vi "Flush Buffer.vi"(0 "VISA resource name":refnum<visa-resource-name>, 7 "milliseconds to wait":u32, 11 "error in (no error)":errorcluster) -> (4 "VISA resource name out":refnum<visa-resource-name>, 6 "read buffer":string, 8 "return count":u32, 10 "Number of Bytes at Serial Port":u32, 15 "error out":errorcluster)   [LabVIEW 2020]
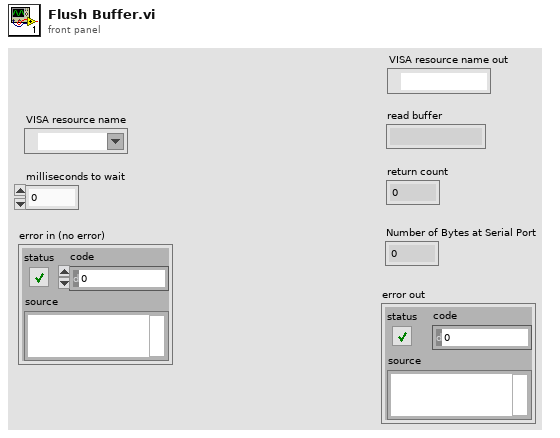
[diagram p1: front panel]
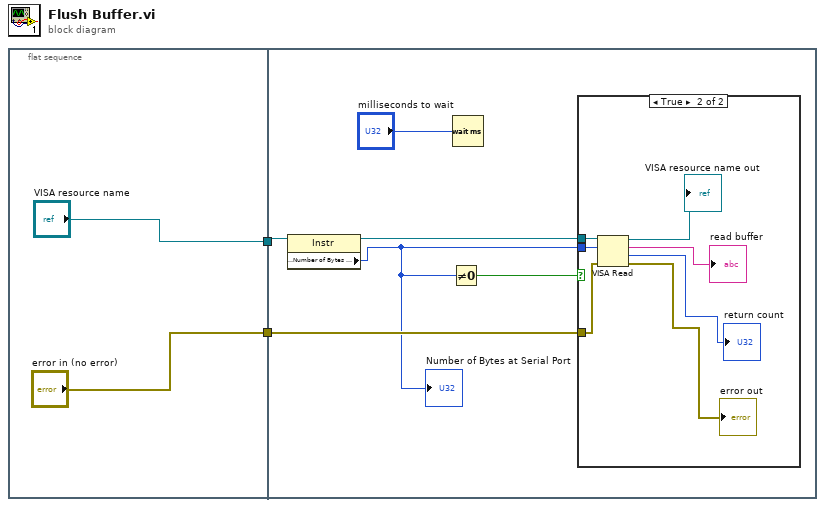
[diagram p0: block diagram]
diagram:
  n1 = flat-sequence {
    tunnel: ["VISA resource name"] -> w2
    tunnel: ["error in (no error)"] -> w1
    tunnel: w1 -> [w10]
    tunnel: w2 -> [w9]
    frame #0 {
    }
    frame #1 {
      n2 = property class="Instr"(reference=w9) -> (reference out=w8:refnum<visa-resource-name>, "Serial Settings:Number of Bytes at Serial Port"=w7:u32)  [unwired: 1 in, 1 out]
      "Number of Bytes at Serial Port" <- w7
      n3 = Not Equal To 0?(x=w7) -> (x != 0?=w6:bool)
      n4 = Wait (ms)(milliseconds to wait="milliseconds to wait") -> ()  [unwired: 1 out]
      n5 = case shown="True" w6 {
        tunnel: w10 -> [_ w13]
        tunnel: w8 -> [_ w12]
        tunnel: w7 -> [_ w11]
        frame False {
        }
        frame True {
          n6 = VISA Read(VISA resource name=w12, byte count=w11, error in (no error)=w13) -> (VISA resource name out=→"VISA resource name out":refnum<visa-resource-name>, read buffer=→"read buffer":string, return count=→"return count":u32, error out=→"error out":errorcluster)
        }
      }
    }
  }
